vi "Agilent 34970 Scale and Setup Voltage.vi"(6 "Channel List":string, 8 "error in (no error)":errorcluster, 9 "Gain (1)":dbl=30.0 format="%#_13g", 11 "VISA Refnum in":refnum<visa-resource-name>) -> (0 "error out":errorcluster, 3 "VISA Refnum out":refnum<visa-resource-name>)   [LabVIEW 2019]
uses:
  Agilent 34970.lvlib
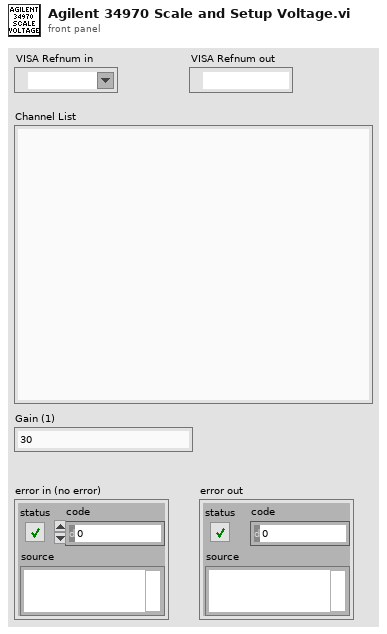
[diagram p1: front panel]
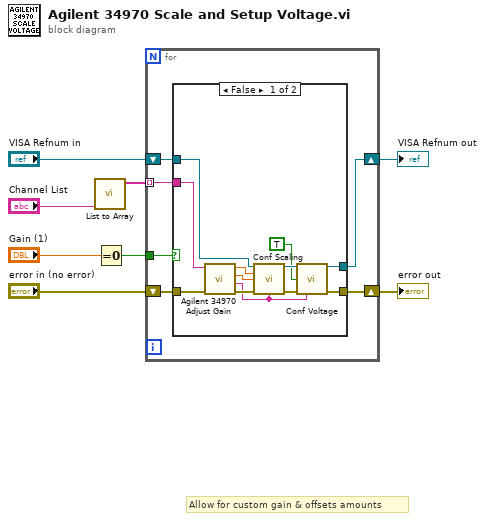
[diagram p0: block diagram]
diagram:
  # "Allow for custom gain & offsets amounts"
  n1 = call "List to Array.vi"("List (empty)"="Channel List") -> ("Output String Array"=w1:string[])  [unwired: 9 in, 1 out]
  n2 = Equal To 0?(x="Gain (1)") -> (x = 0?=w8:bool)
  n3 = for {
    tunnel: w8 -> [w14]
    shift-right: [w12] -> w6
    shift-left: "error in (no error)" -> [w13]
    shift-right: [w10] -> w3
    shift-left: "VISA Refnum in" -> [w11]
    tunnel: w1 -> [w9] mode=indexing
    n4 = case shown="False" w14 {
      tunnel: w13 -> [w19 w28]
      tunnel: [w23 w28] -> w12
      tunnel: w11 -> [w22 w27]
      tunnel: [w21 w27] -> w10
      tunnel: w9 -> [w20 _]
      frame False {
        n5 = call "Agilent 34970 Adjust Gain.vi"("Error In"=w19, "Input Channel"=w20) -> ("Error Out"=w18:errorcluster, "Output Channel"=w15:string, "Offset"=w16:dbl, "Output Gain"=w17:dbl)  [unwired: 5 in, 1 out]
        n6 = call "Conf Scaling.vi"("VISA Resource Name"=w22, "Gain (1)"=w17, "Offset (0)"=w16, "error in (no error)"=w18, "Channel List (empty)"=w15) -> ("VISA Resource Name Out"=w25:refnum<visa-resource-name>, "error out"=w26:errorcluster)  [unwired: 8 in, 1 out]
        n7 = call "Conf Voltage.vi"("VISA Resource Name"=w25, "Autorange? (F:Off)"=TRUE, "error in (no error)"=w26, "Channel List (empty)"=w15) -> ("VISA Resource Name Out"=w21:refnum<visa-resource-name>, "error out"=w23:errorcluster)  [unwired: 9 in, 1 out]
      }
      frame True {
      }
    }
  }
  "error out" <- w6
  "VISA Refnum out" <- w3
